vi "Configure Limits.vi"(6 "Low Limit (0.00)":dbl format="%.2f", 7 "High Limit (10.00)":dbl=10.0 format="%.2f", 8 "error in (no error)":errorcluster, 10 "Enable Limits (True)":bool=TRUE, 11 "VISA resource name":refnum<visa-resource-name>) -> (0 "error out":errorcluster, 3 "VISA resource name out":refnum<visa-resource-name>)   [LabVIEW 2011, in "Fluke 8508.lvlib"]
doc: "This VI enables and sets the limits on the instrument for comparison with each measurement."
uses:
  Fluke 8508.lvlib
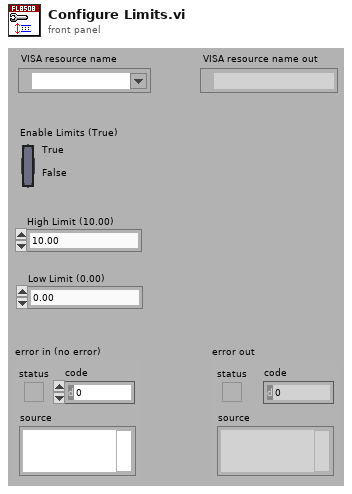
[diagram p1: front panel]
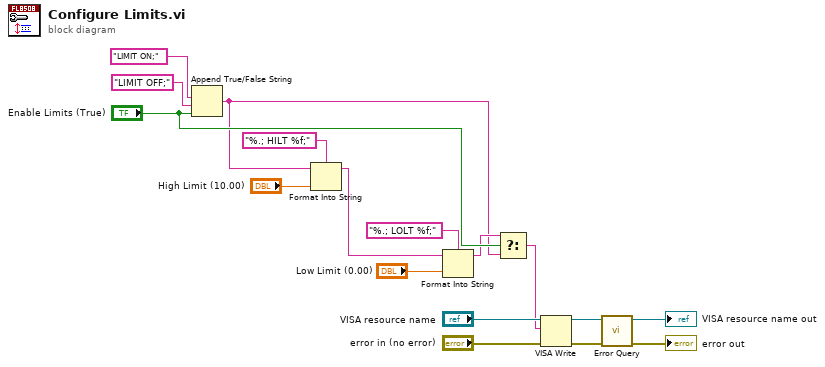
[diagram p0: block diagram]
diagram:
  n1 = Append True/False String(1:"Enable Limits (True)", 2:"LIMIT OFF;" ("false string"), 3:"LIMIT ON;" ("true string")) -> (0:w5:string)  [unwired: 1 in]
  n2 = Format Into String(format string="%.; HILT %f;", initial string=w5, "High Limit (10.00)") -> (resulting string=w9:string)  [unwired: 1 in, 1 out]
  n3 = Format Into String(format string="%.; LOLT %f;", initial string=w9, "Low Limit (0.00)") -> (resulting string=w6:string)  [unwired: 1 in, 1 out]
  n4 = Select(t=w6, s="Enable Limits (True)", f=w5) -> (s? t:f=w8:string)
  n5 = VISA Write(VISA resource name="VISA resource name", write buffer=w8, error in (no error)="error in (no error)") -> (VISA resource name out=w4:refnum<visa-resource-name>, error out=w3:errorcluster)  [unwired: 1 out]
  n6 = call "Error Query.vi"("error in (no error)"=w3, "VISA resource name"=w4) -> ("error out"=→"error out":errorcluster, "VISA resource name out"=→"VISA resource name out":refnum<visa-resource-name>)  [unwired: 6 in, 2 out]
